vi "init ZeroMQ VIs.vi"(8 "error in (no error)":errorcluster, 11 "Header content in":refnum<class "Header content.lvclass">) -> (0 "error out":errorcluster, 3 "Header content out":refnum<class "Header content.lvclass">)   [LabVIEW 2018, in "Header content.lvclass"]
uses:
  Header content.lvclass
  Header content.lvclass/Header content.ctl
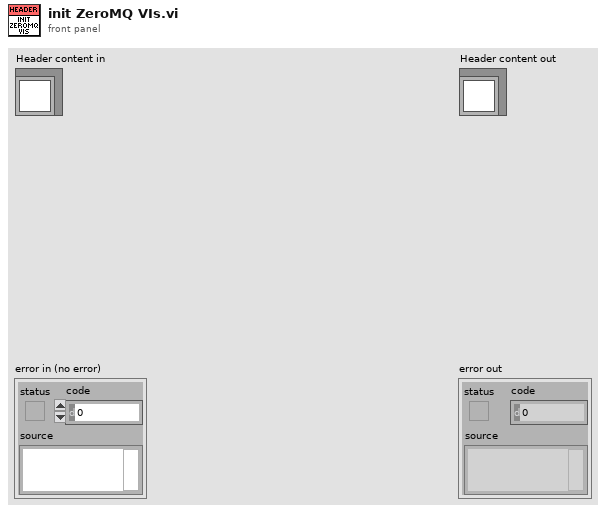
[diagram p1: front panel]
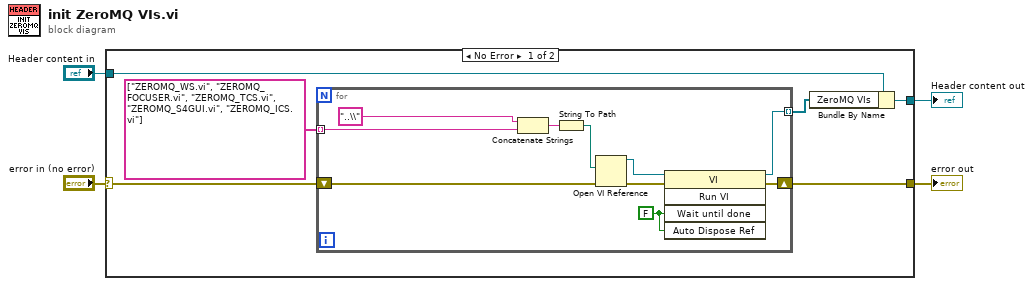
[diagram p0: block diagram]
diagram:
  n1 = case shown="No Error" "error in (no error)" {
    selector: "error in (no error)" -> [w9 w22]
    tunnel: [w8 w22] -> w3
    tunnel: [w6 w21] -> w1
    tunnel: "Header content in" -> [w7 w21]
    frame No Error {
      n2 = for {
        tunnel: string[] ["ZEROMQ_WS.vi", "ZEROMQ_FOCUSER.vi", "ZEROMQ_TCS.vi", "ZEROMQ_S4GUI.vi", "ZEROMQ_ICS.vi"] -> [w16] mode=indexing
        tunnel: [w11] -> w5 mode=indexing
        shift-right: [w12] -> w8
        shift-left: w9 -> [w13]
        w19 = FALSE ("Wait Until Done")
        n3 = Concatenate Strings("..\\", w16) -> (w15:string)
        n4 = String To Path(string=w15) -> (path=w18:path)
        n5 = Open VI Reference(vi path=w18, error in (no error)=w13) -> (vi reference=w20:refnum<vi>, error out=w17:errorcluster)  [unwired: 4 in]
        n6 = invoke class="VI" method="Run VI"(reference=w20, error in=w17, "Wait until done"=w19, "Auto Dispose Ref"=w19) -> (reference out=w11:refnum<vi>, error out=w12:errorcluster)  [unwired: 1 in, 3 out]
      }
      n7 = Bundle By Name(cluster=w7, "ZeroMQ VIs"=w5) -> (w6:refnum<class "Header content.lvclass">)
    }
    frame Error {
    }
  }
  "error out" <- w3
  "Header content out" <- w1
